vi "WSP2_GetDateTimeStr.vi"() -> (0 "Time":string)   [LabVIEW 2017]
uses:
  C:/ClubCar EOL/WSConnector/WSConnector.dll
  WSConnector/WSConnector.dll
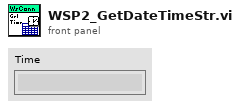
[diagram p1: front panel]
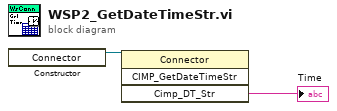
[diagram p0: block diagram]
diagram:
  n1 = constructor class="Connector"() -> (reference out=w2:refnum<k24>)  [unwired: 3 in, 2 out]
  n2 = invoke class="Connector" method="CIMP_GetDateTimeStr"(reference=w2) -> ("Cimp_DT_Str"=→"Time":string)  [unwired: 3 in, 3 out]
